vi "HEXAA INTERVIEW QUESTION Final.vi"() -> ()   [LabVIEW 2020]
panel:
  in  "stop":bool
  out "Numeric 2":i32
  out "Numeric":i32
  in  "Boolean 2":bool
  in  "Boolean":bool
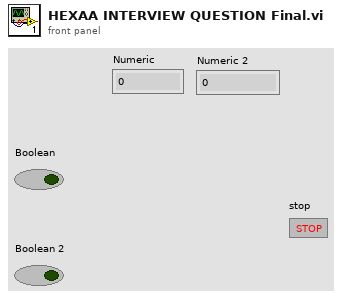
[diagram p1: front panel]
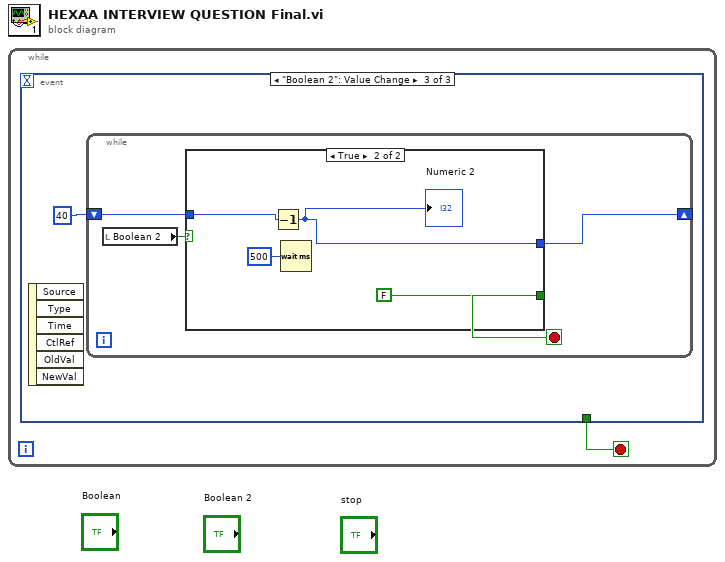
[diagram p0: block diagram]
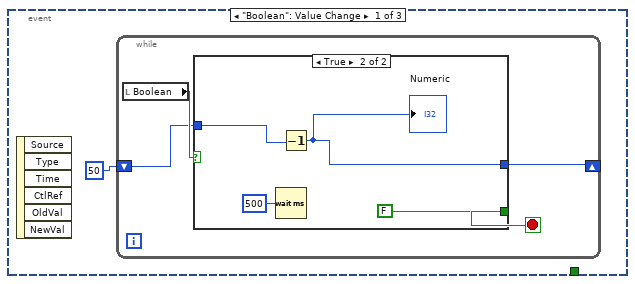
[diagram p2: hidden frame]
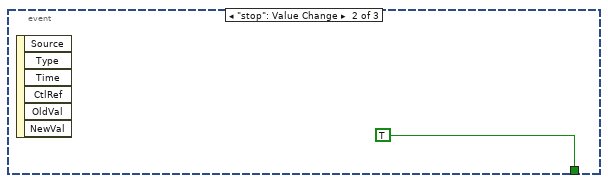
[diagram p4: hidden frame]
diagram:
  n1 = while {
    stop <- w1 stop-if-true
    n2 = event shown="[2] \"Boolean 2\": Value Change" {
      selector: _ -> [_ _ _]
      dyn-events: _ -> [_ _ _]
      timeout: _ -> [_ _ _]
      tunnel: [_ TRUE _] -> w1
      event "Boolean": Value Change {
        n3 = event-data() -> ()  [unwired: 1 in, 6 out]
        n4 = while {
          shift-right: [w3] -> _
          shift-left: 50 -> [w5]
          stop <- w4 stop-if-true
          n5 = local read "Boolean"() -> (w6:bool)
          n6 = case shown="True" w6 {
            tunnel: w5 -> [_ w10]
            tunnel: [_ w9] -> w3
            tunnel: [_ FALSE] -> w4
            frame False {
            }
            frame True {
              n7 = Wait (ms)(milliseconds to wait=u32 500) -> ()  [unwired: 1 out]
              n8 = Decrement(x=w10) -> (x-1=w9:i32)
              "Numeric" <- w9
            }
          }
        }
      }
      event "stop": Value Change {
        n9 = event-data() -> ()  [unwired: 1 in, 6 out]
      }
      event "Boolean 2": Value Change {
        n10 = event-data() -> ()  [unwired: 1 in, 6 out]
        n11 = while {
          shift-right: [w13] -> _
          shift-left: 40 -> [w15]
          stop <- w14 stop-if-true
          n12 = local read "Boolean 2"() -> (w16:bool)
          n13 = case shown="True" w16 {
            tunnel: [_ w20] -> w13
            tunnel: w15 -> [_ w19]
            tunnel: [_ FALSE] -> w14
            frame False {
            }
            frame True {
              n14 = Decrement(x=w19) -> (x-1=w20:i32)
              "Numeric 2" <- w20
              n15 = Wait (ms)(milliseconds to wait=u32 500) -> ()  [unwired: 1 out]
            }
          }
        }
      }
    }
  }
